vi "3 - Event Queue Decoupled from Generation with dotNET PerformanceCounter.vi"() -> ()   [LabVIEW 2012]
panel:
  out "MB used by this VI (appx)":sgl format="%.0f MB"
  in  "Suspend \"B\"":bool
  in  "Suspend \"A\"":bool
  out "Messenger already dead?":errorcluster
  in  "Kill the Messenger":bool
  out "\"B\" already unregistered?":errorcluster
  out "\"A\" already unregistered?":errorcluster
  in  "Register Mailbox \"B\"":bool
  in  "Unregister Mailbox \"B\"":bool
  in  "Unregister Mailbox \"A\"":bool
  in  "Register Mailbox \"A\"":bool
  out "Messages Sent":i32
  in  "stop":bool
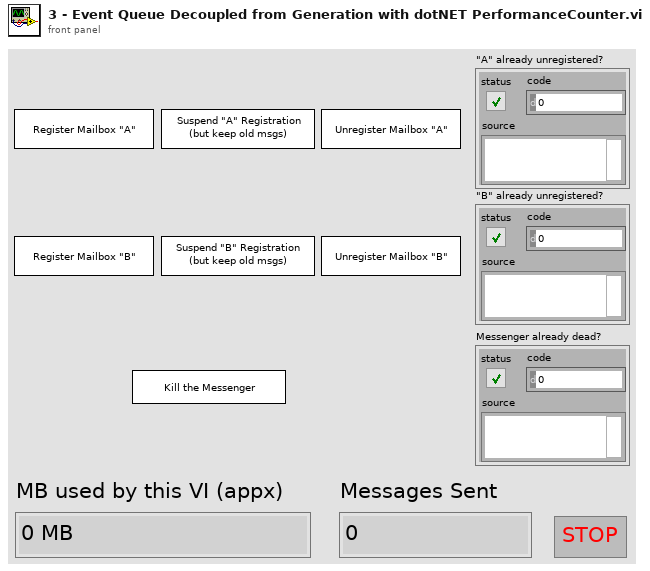
[diagram p1: front panel]
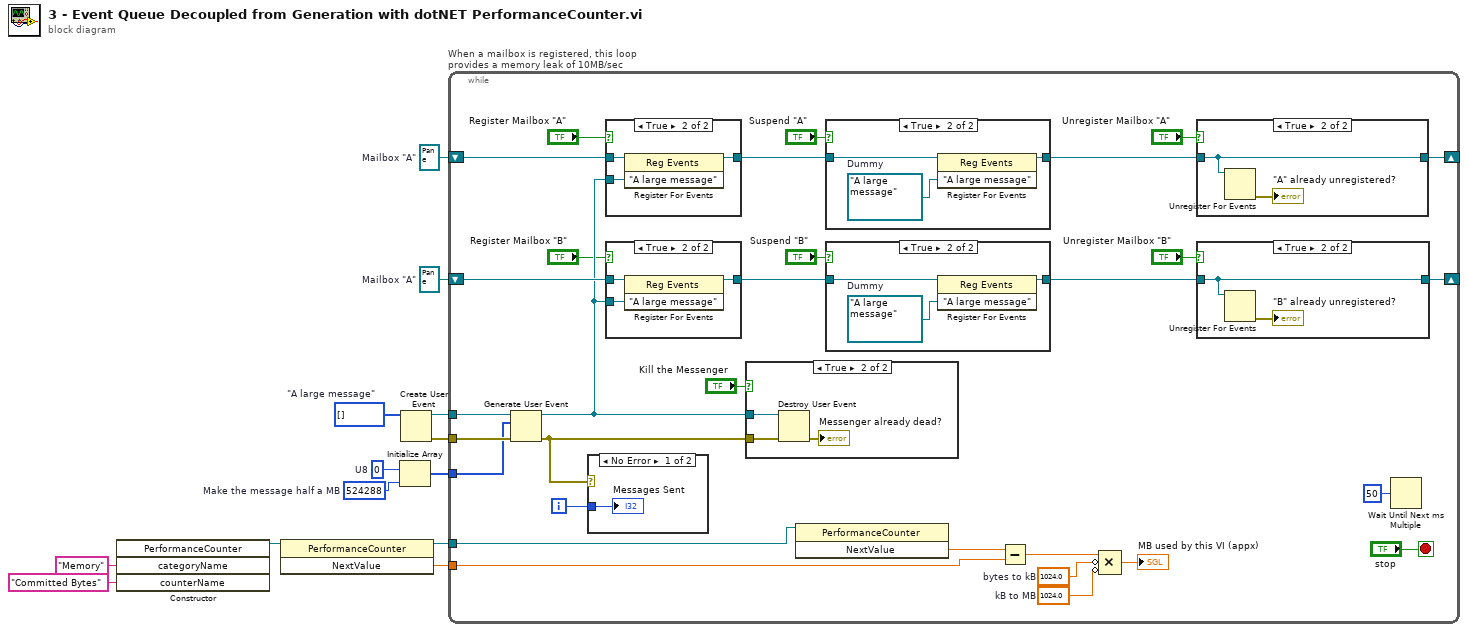
[diagram p0: block diagram]
diagram:
  w6 = refnum<event-registration> refnum  # Mailbox "A"
  w7 = refnum<event-registration> refnum  # Mailbox "A"
  w8 = u8[] []  # "A large message"
  w12 = 524288  # Make the message half a MB
  w13 = u8 0  # U8
  n1 = constructor class="PerformanceCounter"("categoryName"="Memory", "counterName"="Committed Bytes") -> (reference out=w3:refnum<k24>)  [unwired: 3 in, 4 out]
  n2 = invoke class="PerformanceCounter" method="NextValue"(reference=w3) -> (reference out=w2:refnum<k24>, "NextValue"=w1:sgl)  [unwired: 2 in, 1 out]
  n3 = Initialize Array(w13, w12) -> (w9:u8[])
  n4 = Create User Event(user event datatype=w8) -> (user event=w10:refnum<user-event>, error out=w11:errorcluster)  [unwired: 1 in]
  n5 = while "When a mailbox is registered, this loop provides a memory leak of 10MB/sec" {
    tunnel: w11 -> [w42]
    tunnel: w10 -> [w43]
    tunnel: w9 -> [w40]
    shift-right: [w35] -> _
    shift-left: w7 -> [w38]
    shift-right: [w36] -> _
    shift-left: w6 -> [w37]
    tunnel: w2 -> [w20]
    tunnel: w1 -> [w16]
    i -> [w31]
    stop <- "stop" stop-if-true
    w18 = sgl 1024.0  # kB to MB
    w19 = sgl 1024.0  # bytes to kB
    n6 = Generate User Event(user event=w43, event data cluster=w40, error in=w42) -> (user event out=w33:refnum<user-event>, error out=w32:errorcluster)
    n7 = case shown="No Error" w32 {
      tunnel: w31 -> [w52 _]
      frame No Error {
        "Messages Sent" <- w52
      }
      frame Error {
      }
    }
    n8 = case shown="True" "Register Mailbox \"A\"" {
      tunnel: w33 -> [_ w65]
      tunnel: w37 -> [w62 w64]
      tunnel: [w62 w63] -> w28
      frame False {
      }
      frame True {
        n9 = register-events(reference=w64, w65) -> (reference out=w63:refnum<event-registration>)  [unwired: 1 in, 1 out]
      }
    }
    n10 = case shown="True" "Register Mailbox \"B\"" {
      tunnel: w33 -> [_ w69]
      tunnel: w38 -> [w66 w68]
      tunnel: [w66 w67] -> w30
      frame False {
      }
      frame True {
        n11 = register-events(reference=w68, w69) -> (reference out=w67:refnum<event-registration>)  [unwired: 1 in, 1 out]
      }
    }
    n12 = case shown="True" "Kill the Messenger" {
      tunnel: w33 -> [_ w55]
      tunnel: w32 -> [_ w53]
      frame False {
      }
      frame True {
        n13 = Destroy User Event(user event=w55, error in=w53) -> (error out=→"Messenger already dead?":errorcluster)
      }
    }
    n14 = invoke class="PerformanceCounter" method="NextValue"(reference=w20) -> ("NextValue"=w15:sgl)  [unwired: 2 in, 2 out]
    n15 = case shown="True" "Suspend \"A\"" {
      tunnel: w28 -> [w44 w47]
      tunnel: [w44 w46] -> w27
      frame False {
      }
      frame True {
        w45 = refnum<user-event> refnum  # Dummy
        n16 = register-events(reference=w47, w45) -> (reference out=w46:refnum<event-registration>)  [unwired: 1 in, 1 out]
      }
    }
    n17 = case shown="True" "Suspend \"B\"" {
      tunnel: w30 -> [w48 w51]
      tunnel: [w48 w50] -> w29
      frame False {
      }
      frame True {
        w49 = refnum<user-event> refnum  # Dummy
        n18 = register-events(reference=w51, w49) -> (reference out=w50:refnum<event-registration>)  [unwired: 1 in, 1 out]
      }
    }
    n19 = Subtract(x=w15, y=w16) -> (x-y=w14:sgl)
    n20 = Compound Arithmetic op=MULTIPLY(w14, invert w19, invert w18) -> (→"MB used by this VI (appx)":sgl)
    n21 = case shown="True" "Unregister Mailbox \"A\"" {
      tunnel: w27 -> [w59 w61]
      tunnel: [w59 w61] -> w36
      frame False {
      }
      frame True {
        n22 = Unregister For Events(event registration refnum=w61) -> (error out=→"\"A\" already unregistered?":errorcluster)  [unwired: 1 in]
      }
    }
    n23 = case shown="True" "Unregister Mailbox \"B\"" {
      tunnel: w29 -> [w56 w58]
      tunnel: [w56 w58] -> w35
      frame False {
      }
      frame True {
        n24 = Unregister For Events(event registration refnum=w58) -> (error out=→"\"B\" already unregistered?":errorcluster)  [unwired: 1 in]
      }
    }
    n25 = Wait Until Next ms Multiple(millisecond multiple=u32 50) -> ()  [unwired: 1 out]
  }
